vi "74HC162设计一个五进制计数器.vi"() -> ()   [LabVIEW 2018]
panel:
  in  "确定按钮":bool
  out "bit 0":bool
  out "bit1":bool
  out "bit 2":bool
  in  "CLK":bool
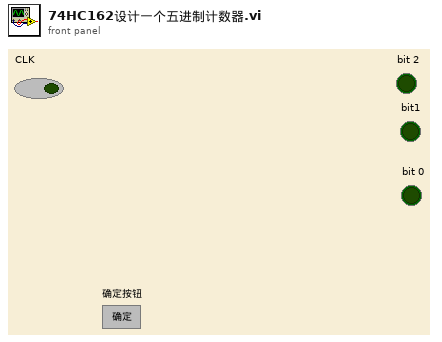
[diagram p1: front panel]
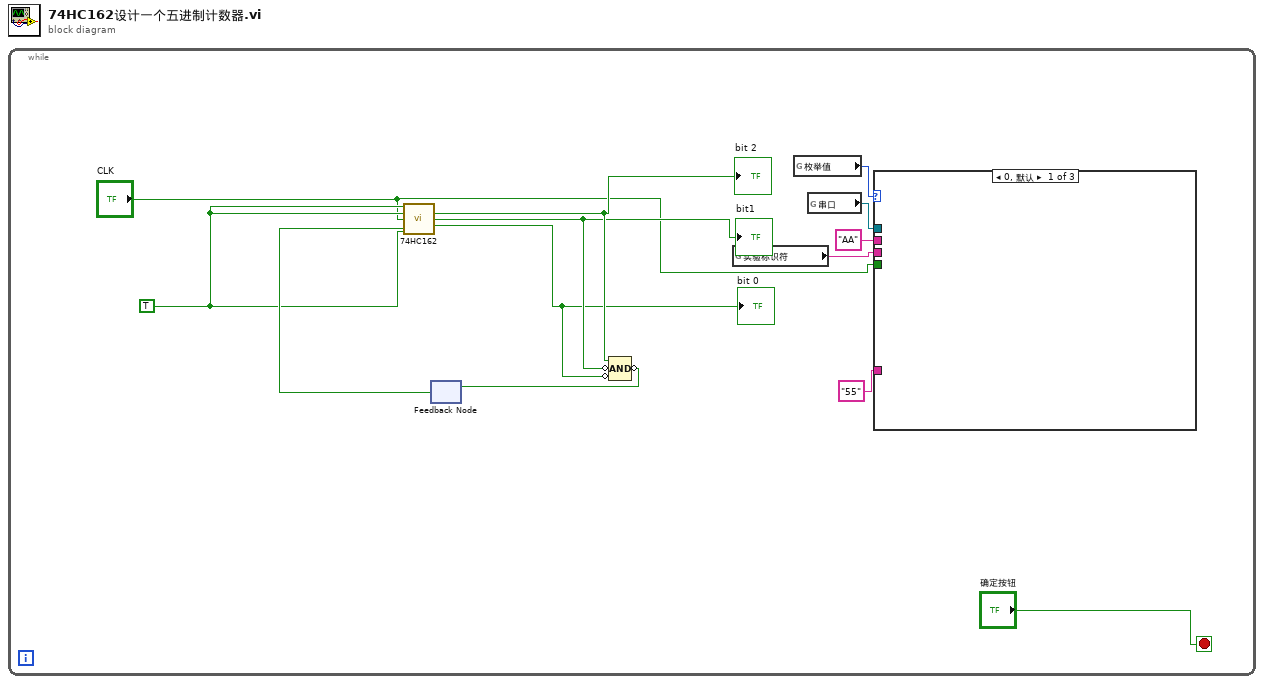
[diagram p0: block diagram]
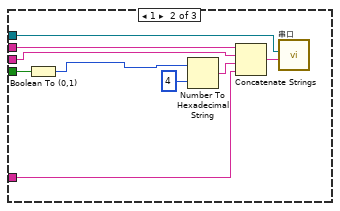
[diagram p2: hidden frame]
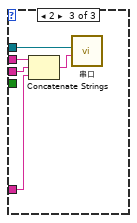
[diagram p3: hidden frame]
diagram:
  n1 = while {
    stop <- "确定按钮" stop-if-true
    w8 = TRUE
    n2 = feedback #1() -> (w9:bool)  [unwired: 1 in]
    n3 = call "74HC162.vi"("EP"=w8, "ET"=w8, "cp"="CLK", "CR`"=w9, "LD`"=w8) -> ("Q2"=w13:bool, "Q1"=w12:bool, "Q0"=w11:bool)  [unwired: 6 in, 2 out]
    "bit 2" <- w13
    "bit1" <- w12
    "bit 0" <- w11
    n4 = Compound Arithmetic op=AND ("复合运算")(w13, invert w12, invert w11) -> (invert w10:bool)
    n5 = feedback-in #1(w10) -> ()
    n6 = global read "全局变量.vi" "实验标识符"() -> (w4:string)
    n7 = global read "全局变量.vi" "枚举值"() -> (w6:i8)
    n8 = global read "全局变量.vi" "串口"() -> (w5:refnum<visa-resource-name>)
    n9 = case shown="0, 默认" w6 {
      tunnel: "CLK" -> [_ w21 _]
      tunnel: w5 -> [_ w20 w25]
      tunnel: w4 -> [_ w19 w26]
      tunnel: "55" -> [_ w18 w23]
      tunnel: "AA" -> [_ w17 w24]
      frame 0, Default {
      }
      frame 1 {
        n10 = Boolean To (0,1)(Boolean=w21) -> (0, 1=w14:i16)
        n11 = Number To Hexadecimal String(1:4, 2:w14) -> (0:w15:string)
        n12 = Concatenate Strings(w17, w19, w15, w18) -> (w22:string)
        n13 = call "串口.vi"("字符串"=w22, "VISA resource name"=w20) -> ()  [unwired: 10 in]
      }
      frame 2 {
        n14 = Concatenate Strings(w24, w26, w23) -> (w27:string)
        n15 = call "串口.vi"("字符串"=w27, "VISA resource name"=w25) -> ()  [unwired: 10 in]
      }
    }
  }
